vi "Initialize.vi"(8 "error in":errorcluster, 10 "shared resources":refnum<class "Shared Resources.lvclass">, 11 "Ballard ARINC-429 Tx Acyclic execution unit in":refnum<class "Tx Acyclic Labels Execution Unit.lvclass">) -> (0 "error out":errorcluster, 3 "Ballard ARINC-429 Tx Acyclic execution unit out":refnum<class "Tx Acyclic Labels Execution Unit.lvclass">)   [LabVIEW 2020, in "Ballard ARINC 429 Engine.lvlib" / "Implementation.lvlib" / "Tx Acyclic Labels Execution Unit.lvclass"]
uses:
  Tx Acyclic Labels Execution Unit.lvclass
  C:/Users/nitest/Desktop/niveristand-ballard-arinc429-custom-device/Source/Custom Device Support/Engine/Implementation/Execution Unit/Execution Unit.lvclass
  Interfaces/Shared Resources/Shared Resources.lvclass
  Shared Resources/Shared Resources.lvclass
  Shared Resources/Shared Resources.lvclass/Shared Resources.ctl
  Execution Unit/Execution Unit.lvclass/Execution Unit.ctl
  Tx Acyclic Labels Execution Unit.lvclass/Tx Acyclic Labels Execution Unit.ctl
  Custom Device/Custom Device.lvlib
  Execution Unit/Execution Unit.lvclass
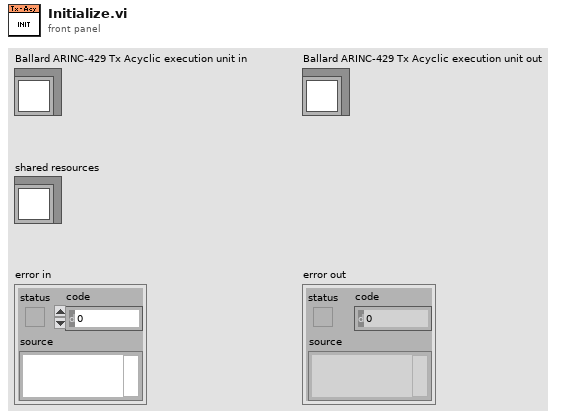
[diagram p1: front panel]
types:
  T1 = typedef "Ballard ARINC 429 Engine.lvlib/Custom Device.lvlib/Hardware Handles.ctl" = cluster{"core handle":u64, "core reader handle":u64, "channel handles":u64[]}
  T2 = typedef "RT Hardware Channel Settings.ctl" = cluster{"channel #":u16, "channel handle":u64, "labels settings for RT":T3[]}
  T3 = typedef "RT Label Settings.ctl" = cluster{"Name":string, "xmlName":string, "label":T4, "transfer period":u32, "SDI_Enabled":bool, "SDI":u8, "parameter driver data":T5, "transfer type":T9, "has timestamp?":bool, "Label Disable/Trigger Channel Reference":T8, "Message Handle":u64, "Initialized?":bool, "Word Initial Raw Value":u32, "Label Timestamp Channel Data Reference":T10, "disabled":bool}
  T4 = typedef "Label.ctl" = u8
  T5 = typedef "RT Parameters.ctl" = cluster{"parameter definitions":T6[], "Tx parameter refs":T8[]}
  T6 = typedef "Parameter Definition.ctl" = cluster{"start index":i32, "size":i32, "encoding":T7, "signed":bool, "scale multiplier":dbl, "scale offset":dbl}
  T7 = typedef "Encoding and Decoding.lvlib/Encoding.ctl" = enum16{"BNR", "BCD", "Discrete"}
  T8 = typedef "Custom Device API.lvlib/Custom Device Item Ref.ctl" = u64
  T9 = typedef "Transfer Type.ctl" = enum16{"Scheduled", "Acyclic", "Block", "Strobe"}
  T10 = typedef "Custom Device API.lvlib/Data Reference.ctl" = i32
  T11 = typedef "Map of Values Indexes to Channel and Label Indexes.ctl" = map{i32, cluster{"channel index":i32, "label index":i32, "group values start index":i32, "values in group":i32}}
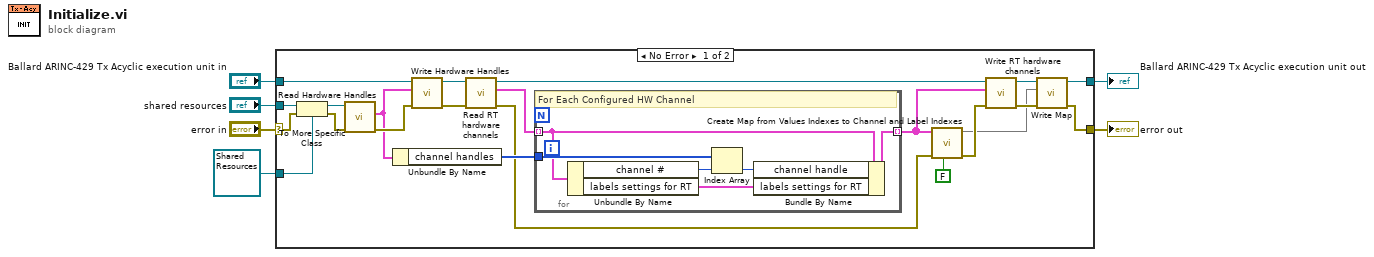
[diagram p0: block diagram]
diagram:
  n1 = case shown="No Error" "error in" {
    selector: "error in" -> [w13 w35]
    tunnel: "Ballard ARINC-429 Tx Acyclic execution unit in" -> [w17 w36]
    tunnel: [w21 w36] -> w5
    tunnel: [w20 w35] -> w3
    tunnel: "shared resources" -> [w11 _]
    tunnel: refnum<class "Shared Resources.lvclass"> refnum ("Ballard ARINC-429 shared resources in") -> [w10 _]
    frame No Error {
      n2 = To More Specific Class(target class=w10, reference=w11, error in=w13) -> (specific class reference=w9:refnum<class "Shared Resources.lvclass">, error out=w12:errorcluster)
      n3 = call "Read Hardware Handles.vi"("error in"=w12, "Ballard ARINC-429 shared resources in"=w9) -> ("error out"=w18:errorcluster, "hardware handles"=w15:T1)  [unwired: 7 in, 1 out]
      n4 = Unbundle By Name(w15) -> ("channel handles"=w28:u64[])
      n5 = call "Write Hardware Handles.vi"("error in"=w18, "hardware handles"=w15, "Ballard ARINC-429 Execution Unit in"=w17) -> ("error out"=w14:errorcluster, "Ballard ARINC-429 Execution Unit out"=w16:refnum<class "Tx Acyclic Labels Execution Unit.lvclass">)  [unwired: 7 in]
      n6 = call "Read RT hardware channels.vi"("error in"=w14, "Ballard ARINC-429 Tx Acyclic execution unit in"=w16) -> ("error out"=w7:errorcluster, "RT hardware channels"=w27:T2[], "Ballard ARINC-429 Tx Acyclic execution unit out"=w26:refnum<class "Tx Acyclic Labels Execution Unit.lvclass">)  [unwired: 7 in]
      n7 = for {
        tunnel: w27 -> [w31] mode=indexing
        tunnel: w28 -> [w33]
        tunnel: [w29] -> w25 mode=indexing
        # "For Each Configured HW Channel"
        n8 = Unbundle By Name(w31) -> ("channel #"=w34:u16, "labels settings for RT"=w30:T3[])
        n9 = Index Array(array=w33, index=w34) -> (element=w32:u64)
        n10 = Bundle By Name(cluster=w31, "channel handle"=w32, "labels settings for RT"=w30) -> (w29:T2)
      }
      n11 = call "Create Map from Values Indexes to Channel and Label Indexes.vi"("disable channel included in group"=FALSE, "error in"=w7, "RT hardware channels"=w25) -> ("error out"=w24:errorcluster, "map from values index to RT info indexes"=w19:T11)  [unwired: 7 in]
      n12 = call "Write RT hardware channels.vi"("error in"=w24, "RT hardware channels"=w25, "Ballard ARINC-429 Tx Acyclic execution unit in"=w26) -> ("error out"=w23:errorcluster, "Ballard ARINC-429 Tx Acyclic execution unit out"=w22:refnum<class "Tx Acyclic Labels Execution Unit.lvclass">)  [unwired: 7 in]
      n13 = call "Write Map.vi"("error in"=w23, "map from values indexes to RT info indexes"=w19, "Ballard ARINC-429 Tx Acyclic execution unit in"=w22) -> ("error out"=w20:errorcluster, "Ballard ARINC-429 Tx Acyclic execution unit out"=w21:refnum<class "Tx Acyclic Labels Execution Unit.lvclass">)  [unwired: 7 in]
    }
    frame Error {
    }
  }
  "error out" <- w3
  "Ballard ARINC-429 Tx Acyclic execution unit out" <- w5
